vi "Insert into Sub Panel.vi"(8 "error in (no error)":errorcluster, 10 "VI Reference":refnum<vi>, 11 "Sub Panel Reference":refnum<vi>) -> (0 "error out":errorcluster)   [LabVIEW 2020]
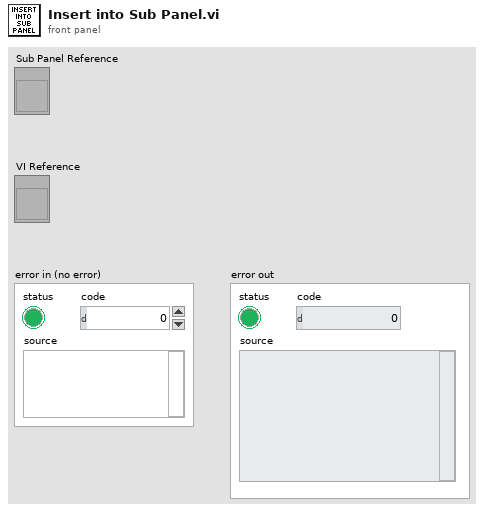
[diagram p1: front panel]
types:
  T1 = enum16{"Always On", "Always Off", "Off While Running"}
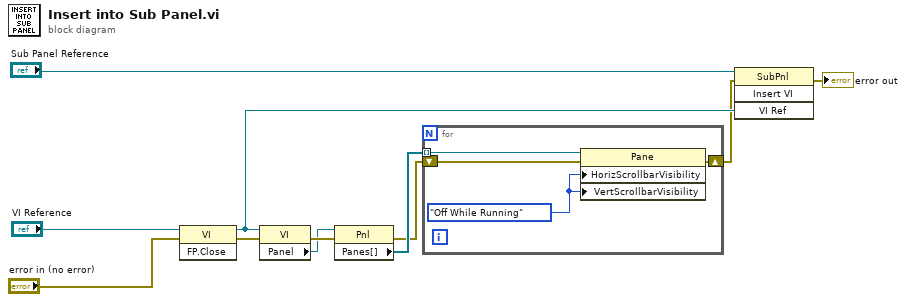
[diagram p0: block diagram]
diagram:
  n1 = invoke class="VI" method="FP.Close"(reference="VI Reference", error in="error in (no error)") -> (reference out=w6:refnum<vi>, error out=w11:errorcluster)  [unwired: 1 in, 1 out]
  n2 = property class="VI"(reference=w6, error in=w11) -> (error out=w10:errorcluster, "Panel"=w7:refnum<vi>)  [unwired: 1 out]
  n3 = property class="Pnl"(reference=w7, error in=w10) -> (error out=w8:errorcluster, "Panes[]"=w9:refnum<vi>[])  [unwired: 1 out]
  n4 = for {
    tunnel: w9 -> [w15] mode=indexing
    shift-right: [w12] -> w5
    shift-left: w8 -> [w13]
    w14 = T1."Off While Running" ("Horizontal Scrollbar Visibility")
    n5 = property class="Pane"(reference=w15, error in=w13, "HorizScrollbarVisibility"=w14, "VertScrollbarVisibility"=w14) -> (error out=w12:errorcluster)  [unwired: 1 out]
  }
  n6 = invoke class="SubPnl" method="Insert VI"(reference="Sub Panel Reference", error in=w5, "VI Ref"=w6) -> (error out=→"error out":errorcluster)  [unwired: 1 in, 3 out]
